vi "finishGoalKickEnemyPlayVSS.vi"(8 "error in (no error)":errorcluster, 10 "Game in":refnum<class "Game.lvclass">, 11 "GoalKickEnemyPlayVSS in":refnum<class "GoalKickEnemyPlayVSS.lvclass">) -> (0 "error out":errorcluster, 2 "result":bool, 3 "GoalKickEnemyPlayVSS out":refnum<class "GoalKickEnemyPlayVSS.lvclass">)   [LabVIEW 2023, in "GoalKickEnemyPlayVSS.lvclass"]
uses:
  GoalKickEnemyPlayVSS.lvclass
  Game_class/Game.lvclass
  Game_class/Game.lvclass/Game.ctl
  Object_class/Object.lvclass/Object.ctl
  Game_class/Read Referee.vi
  Game_class/Read BallRef.vi
  Game_class/Read FieldRef.vi
  Object_class/Read x.vi
  Ball_class/Ball.lvclass
  Referee_class/Referee.lvclass
  Field_class/Field.lvclass
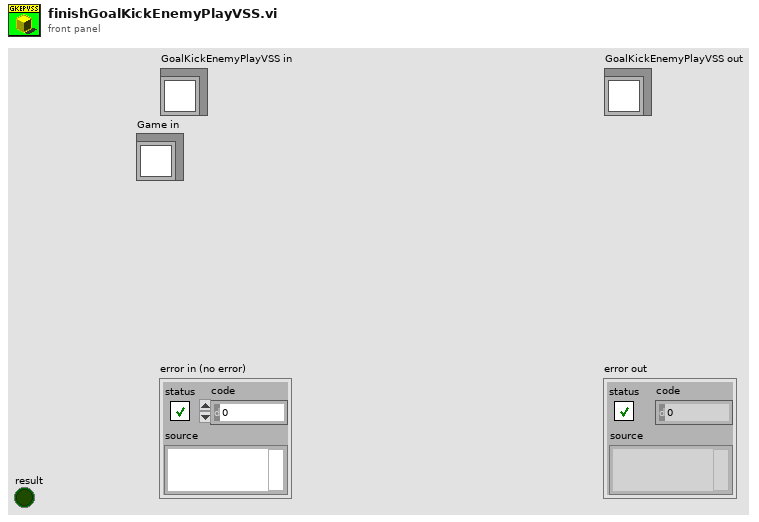
[diagram p1: front panel]
types:
  T1 = enum16{"AUTO", "GAME_ON", "STOP", "KICKOFF", "FREE_BALL", "GOAL_KICK", "PENALTY_KICK", "FREE_KICK"}
  T2 = typedef "Command.ctl" = enum16{"AUTO", "GAME_ON", "STOP", "HALT", "KICKOFF_ALLY", "KICKOFF_ENEMY", "FREE_BALL", "GOAL_KICK_ENEMY", "GOAL_KICK_ALLY", "PENALTY_KICK_ENEMY", "PENALTY_KICK_ALLY", "FREE_KICK"}
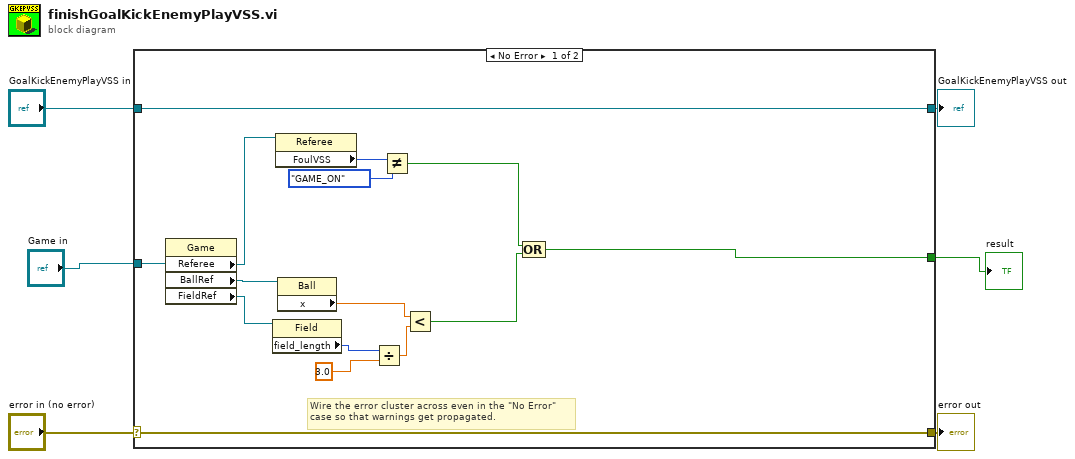
[diagram p0: block diagram]
diagram:
  n1 = case shown="No Error" "error in (no error)" {
    selector: "error in (no error)" -> [w20 w23]
    tunnel: [w20 w23] -> w5
    tunnel: [w21 w22] -> w3
    tunnel: "GoalKickEnemyPlayVSS in" -> [w21 w22]
    tunnel: "Game in" -> [w18 _]
    tunnel: [w17 _] -> w1
    frame No Error {
      # "Wire the error cluster across even in the \"No Error\"\ncase so that warnings get propagated."
      n2 = property class="Game"(reference=w18) -> ("Referee"=w14:refnum<class "Referee.lvclass">, "BallRef"=w19:refnum<class "Ball.lvclass">, "FieldRef"=w12:refnum<class "Field.lvclass">)  [unwired: 1 in, 2 out]
      n3 = property class="Field"(reference=w12) -> ("field_length"=w11:i32)  [unwired: 1 in, 2 out]
      n4 = property class="Referee"(reference=w14) -> ("FoulVSS"=w16:T2)  [unwired: 1 in, 2 out]
      n5 = property class="Ball"(reference=w19) -> ("x"=w8:dbl)  [unwired: 1 in, 2 out]
      n6 = Divide(x=w11, y=3.0) -> (x/y=w9:dbl)
      n7 = Not Equal?(x=w16, y=T1."GAME_ON") -> (x != y?=w13:bool)
      n8 = Less?(x=w8, y=w9) -> (x < y?=w7:bool)
      n9 = Compound Arithmetic op=OR(w13, w7) -> (w17:bool)
    }
    frame Error {
    }
  }
  "error out" <- w5
  "GoalKickEnemyPlayVSS out" <- w3
  "result" <- w1
